vi "prepare_label.vi"(8 "error_in":errorcluster, 11 "reload_active?":bool) -> (0 "error_out":errorcluster, 3 "label_fields":T1)   [LabVIEW 2019]
uses:
  PRINTER/DOCK_PRINTER_label_fields.ctl
  FGV/DOCK_records_display/DOCK_reference_data.ctl
  FGV/DOCK_records_display/FGV_DOCK_records_display.ctl
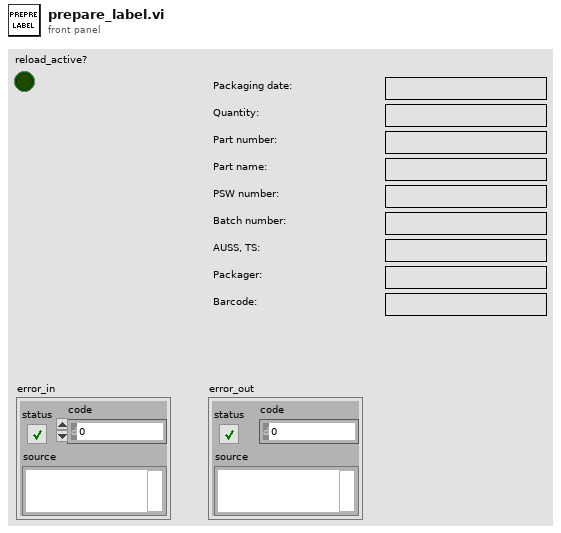
[diagram p1: front panel]
types:
  T1 = typedef "DOCK_PRINTER_label_fields.ctl" = cluster{"packaging_date":string, "quantity":string, "part_number":string, "part_name":string, "PSW_number":string, "batch_number":string, "AUSS, TS":string, "packager":string, "barcode":string}
  T2 = typedef "FGV_DOCK_records_display.ctl" = enum16{"initialize", "set_reference_data", "set_serial", "set_header", "set_operations", "set_results", "set_batches", "get_reference_data", "get_part_number_ref", "get_serial", "get_batch_code", "get_gear_ID", "get_operation_IDs", "toggle_results", "show_all_results", "hide_all_results", "display", "clear"}
  T3 = typedef "DOCK_reference_data.ctl" = cluster{"part_number_ref":string, "part_name_ref":string, "PSW_ref":string, "AUSS_ref":string}
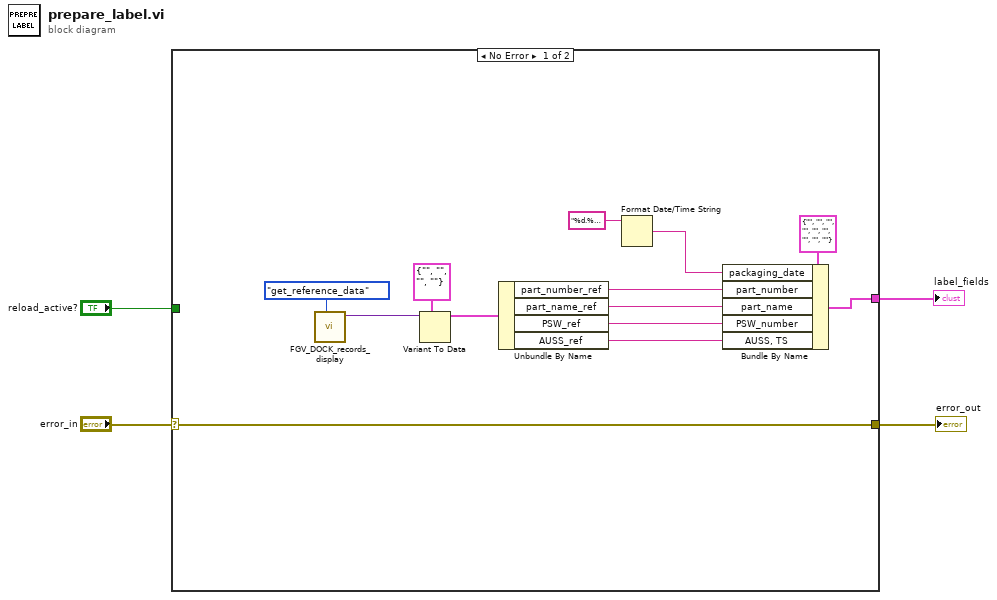
[diagram p0: block diagram]
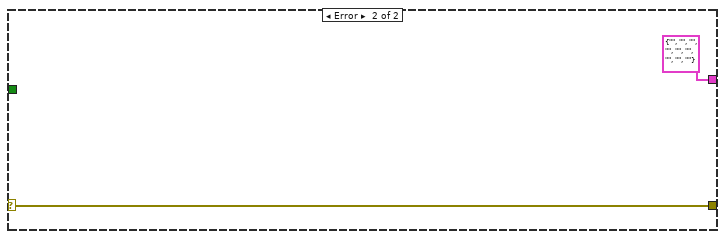
[diagram p2: hidden frame]
diagram:
  n1 = case shown="No Error" "error_in" {
    selector: "error_in" -> [w15 w19]
    tunnel: [w15 w19] -> w3
    tunnel: [w16 T1 {"packaging_date"="", "quantity"="", "part_number"="", "part_name"="", "PSW_number"="", "batch_number"="", "AUSS, TS"="", "packager"="", "barcode"=""} ("label_fields")] -> w2
    tunnel: "reload_active?" -> [_ _]
    frame No Error {
      n2 = call "FGV_DOCK_records_display.vi"("options"=FGV_DOCK_records_display."get_reference_data") -> ("output"=w11:variant)  [unwired: 9 in, 1 out]
      n3 = Variant To Data(type=T3 {"part_number_ref"="", "part_name_ref"="", "PSW_ref"="", "AUSS_ref"=""} ("reference_data"), Variant=w11) -> (data=w9:T3)  [unwired: 1 in, 1 out]
      n4 = Unbundle By Name(w9) -> ("part_number_ref"=w8:string, "part_name_ref"=w7:string, "PSW_ref"=w6:string, "AUSS_ref"=w5:string)
      n5 = Format Date/Time String(time format string (%c)="%d.%m.%Y") -> (date/time string=w13:string)  [unwired: 2 in]
      n6 = Bundle By Name(cluster=T1 {"packaging_date"="", "quantity"="", "part_number"="", "part_name"="", "PSW_number"="", "batch_number"="", "AUSS, TS"="", "packager"="", "barcode"=""} ("label_fields"), "packaging_date"=w13, "part_number"=w8, "part_name"=w7, "PSW_number"=w6, "AUSS, TS"=w5) -> (w16:T1)
    }
    frame Error {
    }
  }
  "error_out" <- w3
  "label_fields" <- w2
